vi "Blink.vi"(8 "error in (no error)":errorcluster, 11 "EPU452 in":refnum<class "EPU452.lvclass">) -> (0 "error out":errorcluster, 3 "EPU452 out":refnum<class "EPU452.lvclass">)   [LabVIEW 2018, in "EPU452.lvclass"]
uses:
  EPU452.lvclass
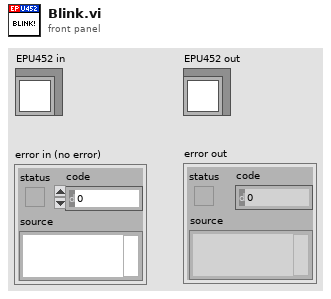
[diagram p1: front panel]
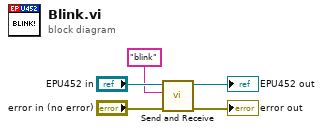
[diagram p0: block diagram]
diagram:
  n1 = call "Send and Receive.vi"("error in (no error)"="error in (no error)", "Command"="blink" ("write buffer"), "EPU452 in"="EPU452 in") -> ("error out"=→"error out":errorcluster, "EPU452 out"=→"EPU452 out":refnum<class "EPU452.lvclass">)  [unwired: 6 in, 1 out]
